vi "shift_send&receive.vi"(8 "error in":errorcluster, 9 "shift string":string=":\u0005\u0000\u0000\u0000\u001f\u0000", 10 "ip address":string=":\u0005\u0000\u0000\u0000\u001f\u0000", 11 "port":refnum<k16>) -> (0 "error out":errorcluster, 3 "connection ID 2":refnum<k16>)   [LabVIEW 2017]
panel:
  out "字符串 4":string
  out "字符串 3":string
  out "data out 3":string="hift"
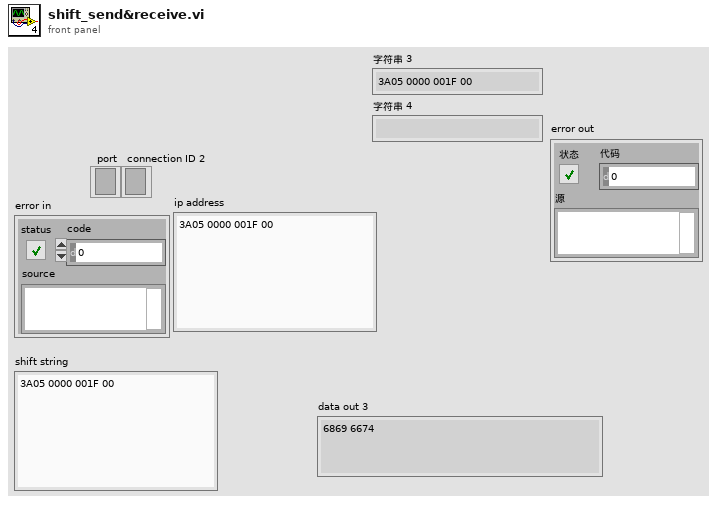
[diagram p1: front panel]
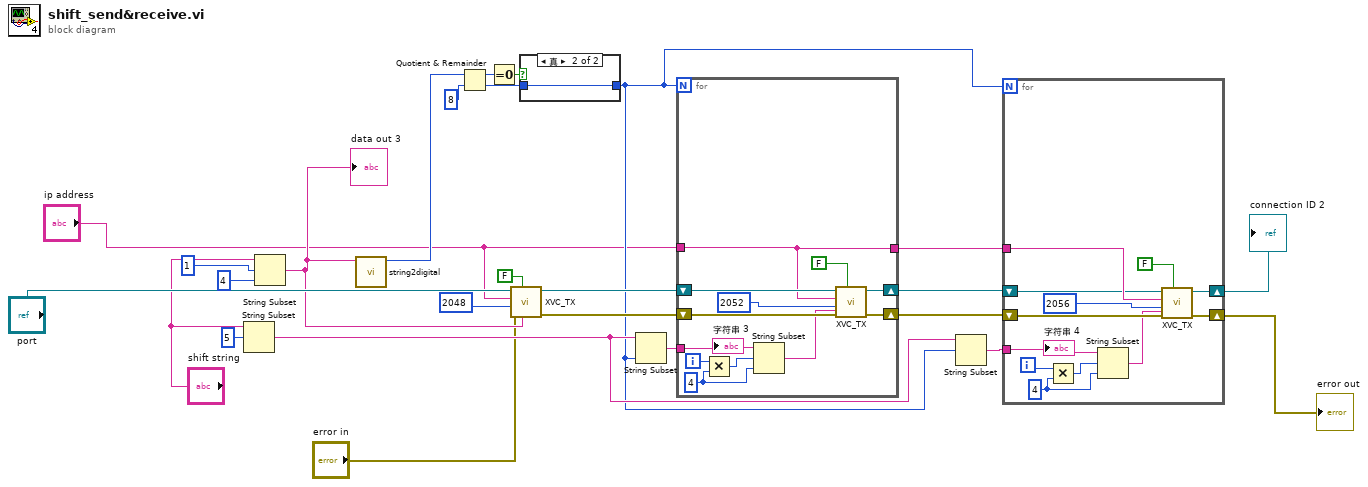
[diagram p0: block diagram]
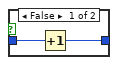
[diagram p2: hidden frame]
diagram:
  n1 = String Subset(string="shift string", offset (0)=5 ("偏移量(0)")) -> (substring=w5:string)  [unwired: 1 in]
  n2 = String Subset(string="shift string", offset (0)=1 ("length (rest)"), length (rest)=4 ("length (rest)")) -> (substring=w12:string)
  "data out 3" <- w12
  n3 = call "string2digital.vi"("data in"=w12) -> ("number"=w26:u32)  [unwired: 10 in]
  n4 = Quotient & Remainder(x=w26, y=u8 8) -> (x-y*floor(x/y)=w20:u32, floor(x/y)=w22:u32)
  n5 = Equal To 0?(x=w20) -> (x = 0?=w21:bool)
  n6 = call "XVC_TX.vi"("data in"=w12, "Read (TRUE)"=FALSE, "error in"="error in", "Address"=u32 2048, "IP address"="ip address", "connection ID"="port") -> ("error out"=w17:errorcluster, "connection ID 2"=w18:refnum<k16>)  [unwired: 3 in, 1 out]
  n7 = case shown="真" w21 {
    tunnel: [w28 w29] -> w4
    tunnel: w22 -> [w27 w29]
    frame False {
      n8 = Increment(x=w27) -> (x+1=w28:u32)
    }
    frame True {
    }
  }
  n9 = String Subset(string=w5, length (rest)=w4) -> (substring=w11:string)  [unwired: 1 in]
  n10 = for {
    N: w4 -> [_]
    tunnel: "ip address" -> [w36]
    shift-right: [w40] -> w9
    shift-left: w17 -> [w41]
    shift-right: [w38] -> w10
    shift-left: w18 -> [w39]
    tunnel: w11 -> [w31]
    tunnel: [w36] -> w7
    i -> [w33]
    w32 = 4 ("长度（剩余）")
    n11 = Multiply(x=w33, y=w32) -> (x*y=w34:i32)
    n12 = String Subset(string=w31, offset (0)=w34, length (rest)=w32) -> (substring=w30:string)
    n13 = call "XVC_TX.vi"("data in"=w30, "Read (TRUE)"=FALSE, "error in"=w41, "Address"=u32 2052, "IP address"=w36, "connection ID"=w39) -> ("error out"=w40:errorcluster, "connection ID 2"=w38:refnum<k16>)  [unwired: 3 in, 1 out]
    "字符串 3" <- w31
  }
  n14 = String Subset(string=w5, offset (0)=w4) -> (substring=w6:string)  [unwired: 1 in]
  n15 = for {
    N: w4 -> [_]
    tunnel: w7 -> [w53]
    shift-right: [w51] -> w3
    shift-left: w9 -> [w52]
    shift-right: [w49] -> w8
    shift-left: w10 -> [w50]
    tunnel: w6 -> [w42]
    i -> [w44]
    w45 = 4 ("长度（剩余）")
    n16 = Multiply(x=w44, y=w45) -> (x*y=w46:i32)
    n17 = String Subset(string=w42, offset (0)=w46, length (rest)=w45) -> (substring=w43:string)
    n18 = call "XVC_TX.vi"("data in"=w43, "Read (TRUE)"=FALSE, "error in"=w52, "Address"=u32 2056, "IP address"=w53, "connection ID"=w50) -> ("error out"=w51:errorcluster, "connection ID 2"=w49:refnum<k16>)  [unwired: 3 in, 1 out]
    "字符串 4" <- w42
  }
  "connection ID 2" <- w8
  "error out" <- w3
